vi "QueueStatus.vi"(8 "error in":errorcluster, 10 "Return Elements? (F)":bool, 11 "PriorityMessageQueue in":refnum<class "PriorityMessageQueue.lvclass">) -> (0 "error out":errorcluster, 1 "# Pending Insert":i32[](array[numeric]), 2 "# Pending Remove":i32[](array[numeric]), 3 "PriorityMessageQueue out":refnum<class "PriorityMessageQueue.lvclass">, 4 "# Elements in Queue":i32[](array[numeric]), 6 "Elements":refnum<class "Message.lvclass">[][](array[class]), 7 "Max Queue Size":i32)   [LabVIEW 2009, in "LapDog.Messaging.v2.lvlib" / "PriorityMessageQueue.lvclass"]
doc: "<b>This class is deprecated in version 2.1 and will be removed in version 3.0</b>\n\nReturns information about the state of the priority queue. Data is returned in arrays with each element in the arrays corresponding to the priority level of the same number. This vi can be used to test if the queue has a valid refnum. If the refnum is invalid error 1 will be returned."
uses:
  PriorityMessageQueue.lvclass
  MessageObject/Message.lvclass
  PriorityMessageQueue.lvclass/PriorityMessageQueue.ctl
panel:
  out "queue name":string
  # "Queue Name has been disconnected from the front panel while I figure out how to best implement a named priority queue."
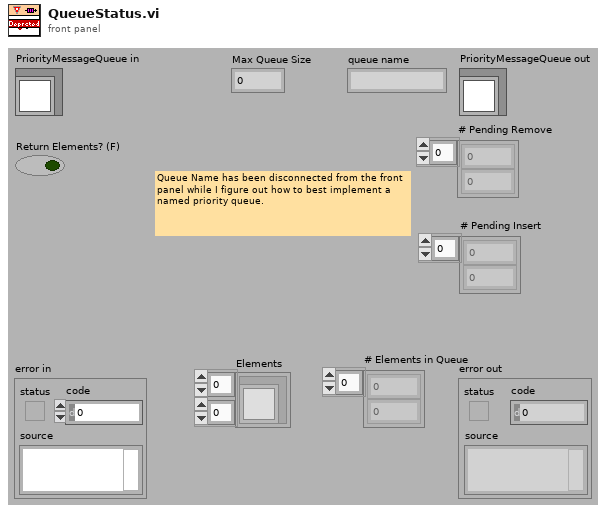
[diagram p1: front panel]
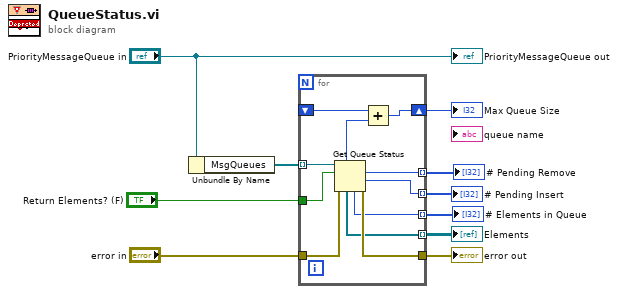
[diagram p0: block diagram]
diagram:
  n1 = Unbundle By Name("PriorityMessageQueue in") -> ("MsgQueues"=w9:refnum<queue>[])
  n2 = for {
    tunnel: w9 -> [w21] mode=indexing
    tunnel: "error in" -> [w20]
    tunnel: [w19] -> w7
    tunnel: "Return Elements? (F)" -> [w18]
    tunnel: [w17] -> w4 mode=indexing
    tunnel: [w16] -> w3 mode=indexing
    tunnel: [w15] -> w2 mode=indexing
    tunnel: [w14] -> w1 mode=indexing
    shift-right: [w12] -> w5
    shift-left: _ -> [w11]
    n3 = Get Queue Status(queue=w21, return elements? (F)=w18, error in (no error)=w20) -> (max queue size=w13:i32, # pending remove=w17:i32, # pending insert=w16:i32, error out=w19:errorcluster, # elements in queue=w15:i32, elements=w14:refnum<class "Message.lvclass">[])  [unwired: 2 out]
    n4 = Add(x=w11, y=w13) -> (x+y=w12:i32)
  }
  "error out" <- w7
  "Max Queue Size" <- w5
  "Elements" <- w1
  "# Pending Remove" <- w4
  "# Pending Insert" <- w3
  "# Elements in Queue" <- w2
  "PriorityMessageQueue out" <- "PriorityMessageQueue in"
